vi "Get Help.vi"(0 "Display State In":T1={"Current Channels Info"=[], "Help Prefix"="", "Max Display Size"=8, "Max Size"=0, "Show Buttons"=TRUE, "Data Valid"=refnum, "Show Range"=FALSE, "Range Items"=[], "Range Index"=[]}, 9 "Container State":T4, 11 "error in (no error)":errorcluster) -> (4 "Display State Out":T1={"Current Channels Info"=[], "Help Prefix"="", "Max Display Size"=8, "Max Size"=0, "Show Buttons"=TRUE, "Data Valid"=refnum, "Show Range"=FALSE, "Range Items"=[], "Range Index"=[]}, 6 "Help":string, 15 "error out":errorcluster)   [LabVIEW 2021, in "myRIO Channel List.xctl"]
uses:
  <vilib>/myRIO/Common/Express VI Framework/xctls/myRIO Channel List/myRIO Channel List.xctl
  <vilib>/_xctls/Container State.ctl
  <vilib>/myRIO/Common/Express VI Framework/xctls/myRIO Channel List/State.ctl
  <vilib>/myRIO/Common/Profile Manager Framework/typedefs/Channel Info.ctl
  <vilib>/myRIO/Common/Express VI Framework/typedefs/Data Validate Ref.ctl
  <vilib>/myRIO/Common/Express VI Framework/xctls/myRIO Channel List/Data.ctl
  <vilib>/myRIO/Common/Express VI Framework/xctls/myRIO Channel List/typedefs/Channel Data.ctl
  <vilib>/myRIO/Common/Express VI Framework/xctls/myRIO Channel List/typedefs/Remove Channel.ctl
  <vilib>/_xctls/XControlSupport.lvlib
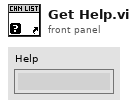
[diagram p1: front panel]
types:
  T1 = typedef "myRIO Channel List.xctl/State.ctl" = cluster{"Current Channels Info":T2[], "Help Prefix":string, "Max Display Size":i32, "Max Size":i32, "Show Buttons":bool, "Data Valid":T3, "Show Range":bool, "Range Items":string[], "Range Index":i32[]}
  T2 = typedef "Channel Info.ctl" = cluster{"Channel Name":string, "Alias":string, "Used?":bool, "Not Support?":bool, "Property Bundle":cluster{"Name":string, "Value":variant}[]}
  T3 = typedef "Data Validate Ref.ctl" = refnum<user-event>
  T4 = typedef "XControlSupport.lvlib/Container State.ctl" = cluster{"Indicator?":bool, "Run Mode?":bool, " Refnum":refnum<vi>}
  T5 = typedef "myRIO Channel List.xctl/Data.ctl" = T6[]
  T6 = typedef "myRIO Channel List.xctl/Channel Data.ctl" = cluster{"Channel Name":u16, "Channel Alias":string, "Remove Channel":T7, "Index":i32}
  T7 = typedef "myRIO Channel List.xctl/Remove Channel.ctl" = bool
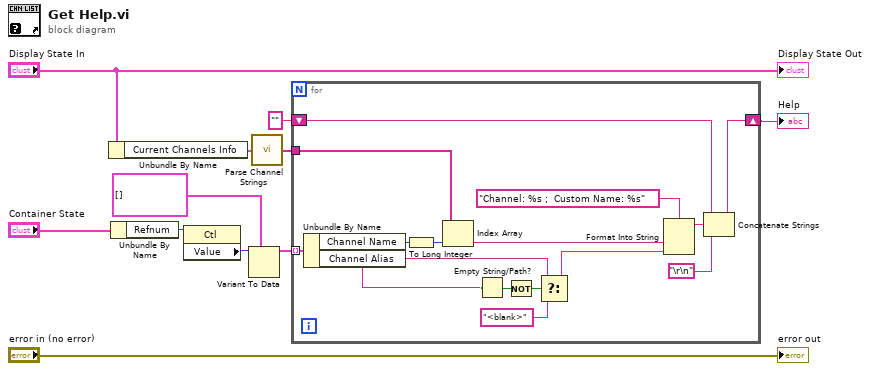
[diagram p0: block diagram]
diagram:
  n1 = Unbundle By Name("Display State In") -> ("Current Channels Info"=w3:T2[])
  n2 = Unbundle By Name("Container State") -> ("Refnum"=w10:refnum<vi>)
  n3 = property class="Ctl"(reference=w10) -> ("Value"=w9:variant)  [unwired: 1 in, 2 out]
  n4 = Variant To Data(type=T5 [] ("Channel List"), Variant=w9) -> (data=w6:T5)  [unwired: 1 in, 1 out]
  n5 = call <vilib>:"Parse Channel Strings.vi"("Channels Info"=w3) -> ("Channel Strings"=w2:string[])
  n6 = for {
    tunnel: w6 -> [w26] mode=indexing
    shift-right: [w14] -> w1
    shift-left: "" -> [w15]
    tunnel: w2 -> [w25]
    n7 = Unbundle By Name(w26) -> ("Channel Name"=w24:u16, "Channel Alias"=w18:string)
    n8 = To Long Integer(number=w24) -> (32bit integer=w23:i32)
    n9 = Index Array(array=w25, index=w23) -> (element=w21:string)
    n10 = Empty String/Path?(string/path=w18) -> (empty?=w20:bool)
    n11 = Not(x=w20) -> (.not. x?=w19:bool)
    n12 = Select(t=w18, s=w19, f="<blank>") -> (s? t:f=w17:string)
    n13 = Format Into String(format string="Channel: %s ;  Custom Name: %s", w21, w17) -> (resulting string=w13:string)  [unwired: 2 in, 1 out]
    n14 = Concatenate Strings(w15, w13, "\r\n") -> (w14:string)
  }
  "Help" <- w1
  "Display State Out" <- "Display State In"
  "error out" <- "error in (no error)"
